vi "CRYOpen Manual.vi"(11 "appended path":path) -> ()   [LabVIEW 2013]
uses:
  <vilib>/registry/registry.llb/Registry RtKey.ctl
  <vilib>/registry/registry.llb/Registry SAM.ctl
panel:
  in  "error in (no error)":errorcluster
  out "error out":errorcluster
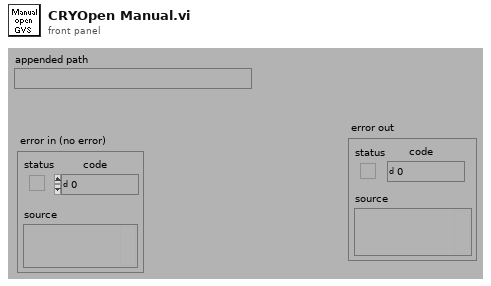
[diagram p1: front panel]
types:
  T1 = typedef "Registry SAM.ctl" = enum32{"KEY_QUERY_VALUE", "KEY_SET_VALUE", "KEY_CREATE_SUB_KEY", "KEY_ENUMERATE_SUB_KEYS", "KEY_NOTIFY", "KEY_CREATE_LINK", "KEY_READ", "KEY_WRITE", "KEY_ALL_ACCESS", "KEY_READ | KEY_WRITE"}
  T2 = typedef "Registry RtKey.ctl" = enum32{"HKEY_CLASSES_ROOT", "HKEY_CURRENT_USER", "HKEY_LOCAL_MACHINE", "HKEY_USERS", "HKEY_PERFORMANCE_DATA", "HKEY_CURRENT_CONFIG", "HKEY_DYN_DATA"}
  T3 = typedef "Registry refnum.ctl" = refnum<k1>
  T4 = cluster{"numValues":i32, "maxValueNameLen":i32, "maxValueDataLen":i32}
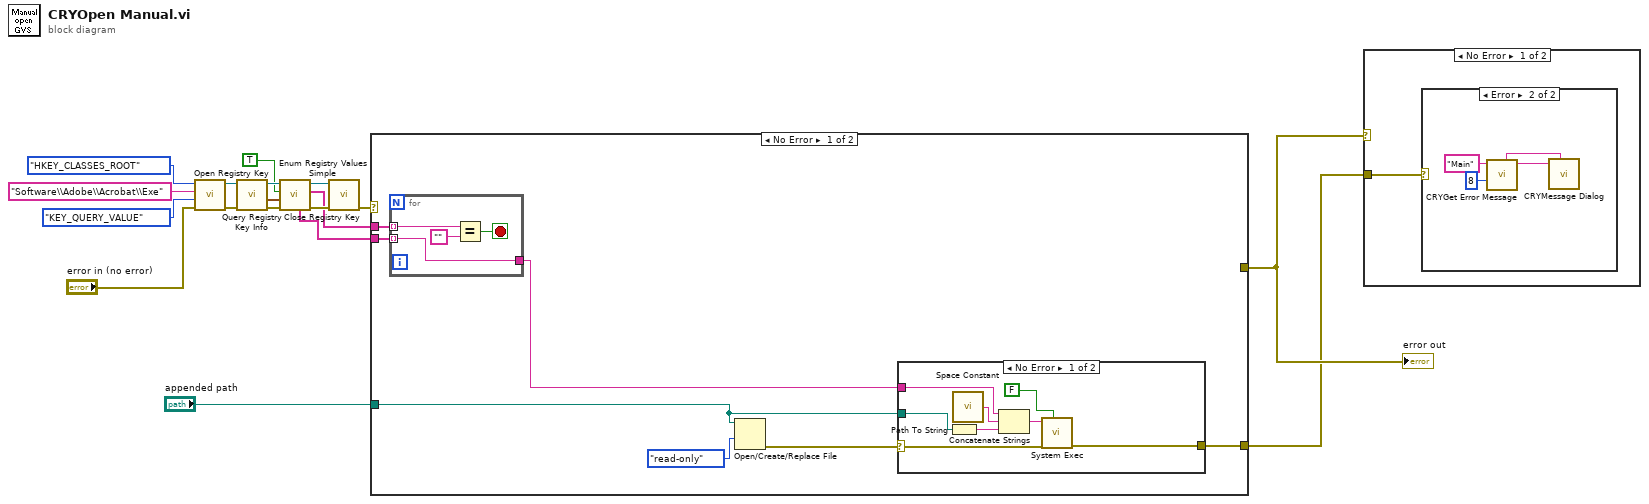
[diagram p0: block diagram]
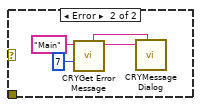
[diagram p3: hidden frame]
diagram:
  n1 = call <vilib>:"Open Registry Key.vi"("error in (no error)"="error in (no error)", "security access mask (KEY_READ | KEY_WRITE)"=Registry_SAM."KEY_QUERY_VALUE", "subkey"="Software\\Adobe\\Acrobat\\Exe", "root key (HKEY_LOCAL_MACHINE)"=Registry_RtKey."HKEY_CLASSES_ROOT") -> ("error out"=w13:errorcluster, "refnum out"=w15:T3)  [unwired: 6 out]
  n2 = call <vilib>:"Query Registry Key Info.vi"("error in (no error)"=w13, "refnum"=w15) -> ("error out"=w12:errorcluster, "value info"=w17:T4, "refnum out"=w16:T3)  [unwired: 7 out]
  n3 = call <vilib>:"Enum Registry Values Simple.vi"("error in (no error)"=w12, "value info"=w17, "retrieve data? (F)"=TRUE, "refnum"=w16) -> ("error out"=w8:errorcluster, "values"=w7:string[], "refnum out"=w18:T3, "String/Binary data"=w6:string[])  [unwired: 4 out]
  n4 = call <vilib>:"Close Registry Key.vi"("error in (no error)"=w8, "refnum"=w18) -> ("error out"=w5:errorcluster)  [unwired: 5 out]
  n5 = case shown="No Error" w5 {
    selector: w5 -> [_ w39]
    tunnel: w7 -> [w25 _]
    tunnel: w6 -> [w24 _]
    tunnel: "appended path" -> [w22 _]
    tunnel: [_ w39] -> w2
    tunnel: [w20 _] -> w1
    frame No Error {
      n6 = for {
        tunnel: w25 -> [w38] mode=indexing
        tunnel: w24 -> [w35] mode=indexing
        tunnel: [w35] -> w19
        stop <- w36 stop-if-true
        n7 = Equal?(x=w38, y="") -> (x = y?=w36:bool)
      }
      n8 = Open/Create/Replace File(file path (use dialog)=w22, access (0:read/write)=enum16{"read/write", "read-only", "write-only"}."read-only") -> (error out=w21:errorcluster)  [unwired: 1 in, 5 out]
      n9 = case shown="No Error" w21 {
        selector: w21 -> [w27 w34]
        tunnel: w19 -> [w29 _]
        tunnel: w22 -> [w28 _]
        tunnel: [w26 w34] -> w20
        frame No Error {
          n10 = Path To String(path=w28) -> (string=w31:string)
          n11 = call <vilib>:"Space Constant.vi"() -> ("String"=w30:string)
          n12 = Concatenate Strings(w29, w30, w31) -> (w32:string)
          n13 = call <vilib>:"System Exec.vi"("wait until completion? (T)"=FALSE, "error in (no error)"=w27, "command line"=w32) -> ("error out"=w26:errorcluster)  [unwired: 3 in, 5 out]
        }
        frame Error {
        }
      }
    }
    frame Error {
    }
  }
  "error out" <- w2
  n14 = case shown="No Error" w2 {
    tunnel: w1 -> [w40 _]
    frame No Error {
      n15 = case shown="Error" w40 {
        frame No Error {
        }
        frame Error {
          n16 = call "CRYGet Error Message.vi"("Error No"=8, "Kind"="Main") -> ("Message"=w43:string, "Window Title"=w44:string)  [unwired: 4 in, 4 out]
          n17 = call "CRYMessage Dialog.vi"("Window Title"=w44, "Message Content"=w43) -> ()  [unwired: 8 in, 2 out]
        }
      }
    }
    frame Error {
      n18 = call "CRYGet Error Message.vi"("Error No"=7, "Kind"="Main") -> ("Message"=w47:string, "Window Title"=w48:string)  [unwired: 4 in, 4 out]
      n19 = call "CRYMessage Dialog.vi"("Window Title"=w48, "Message Content"=w47) -> ()  [unwired: 8 in, 2 out]
    }
  }
